vi "to_json.vi"(8 "error in":errorcluster, 11 "ts.absoloute type in":refnum<class "ts.absoloute type.lvclass">) -> (0 "error out":errorcluster, 2 "json":string, 3 "ts.absoloute type out":refnum<class "ts.absoloute type.lvclass">)   [LabVIEW 2020, in "ts.absoloute type.lvclass"]
uses:
  ts.absoloute type.lvclass
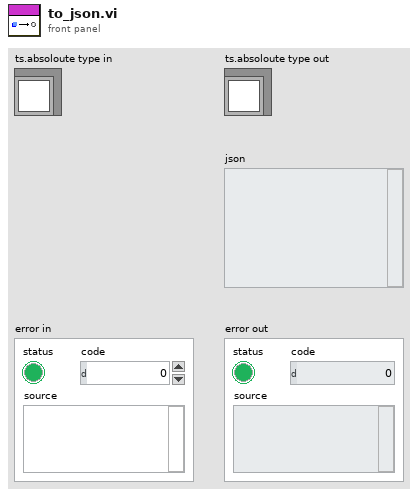
[diagram p1: front panel]
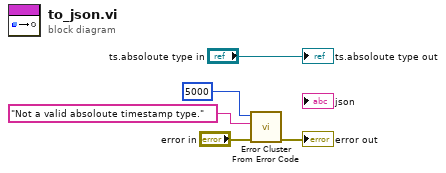
[diagram p0: block diagram]
diagram:
  n1 = call <vilib>:"Error Cluster From Error Code.vi"("error in (no error)"="error in", "error message (\"\")"="Not a valid absoloute timestamp type." ("error message (\"\")"), "error code (0)"=5000) -> ("error out"=→"error out":errorcluster)  [unwired: 6 in]
  "ts.absoloute type out" <- "ts.absoloute type in"
